vi "Replicated Sort.vi"(10 "Panel B":refnum<class "Panel.lvclass">, 11 "Panel A":refnum<class "Panel.lvclass">) -> (3 "A < B":bool)   [LabVIEW 2020, in "SB App.lvlib" / "Dashboard Panel.lvclass"]
uses:
  Dashboard Panel.lvclass
  <vilib>/IlluminatedG/IG OOPanel/OOPanel/Panel/Panel.lvclass
  Team Dashboard Panel/Team Dashboard Panel.lvclass
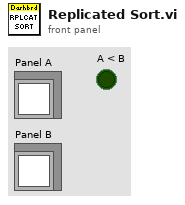
[diagram p1: front panel]
types:
  T1 = typedef "SquareBattle.lvlib/Team Stats.ctl" = cluster{"Squares":i32, "Generated":i32, "Kills":i32, "Eliminated":i32, "Collisions":i32}
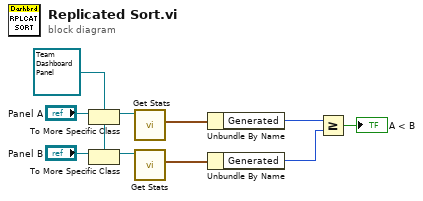
[diagram p0: block diagram]
diagram:
  w8 = refnum<class "Team Dashboard Panel.lvclass"> refnum ("SB App.lvlib:Team Dashboard Panel.lvclass")
  n1 = To More Specific Class(target class=w8, reference="Panel A") -> (specific class reference=w7:refnum<class "Team Dashboard Panel.lvclass">)  [unwired: 1 in, 1 out]
  n2 = To More Specific Class(target class=w8, reference="Panel B") -> (specific class reference=w6:refnum<class "Team Dashboard Panel.lvclass">)  [unwired: 1 in, 1 out]
  n3 = call "Get Stats.vi"("Team Dashboard Panel in"=w7) -> ("Team Stats"=w5:T1)  [unwired: 8 in, 2 out]
  n4 = call "Get Stats.vi"("Team Dashboard Panel in"=w6) -> ("Team Stats"=w4:T1)  [unwired: 8 in, 2 out]
  n5 = Unbundle By Name(w5) -> ("Generated"=w3:i32)
  n6 = Unbundle By Name(w4) -> ("Generated"=w2:i32)
  n7 = Greater Or Equal?(x=w3, y=w2) -> (x >= y?=→"A < B":bool)
